vi "Generate Subpanel to Main Event.vi"(8 "error in (no error)":errorcluster, 9 "data":variant, 10 "command":string, 11 "subpanel to main command event":T1) -> (0 "error out":errorcluster)   [LabVIEW 2017, in "NI_Robotics_Configure Steering Frame.lvlib"]
uses:
  <vilib>/robotics/Dialog/Configure Steering Frame/NI_Robotics_Configure Steering Frame.lvlib
  <vilib>/robotics/Dialog/Configure Steering Frame/Subpanel to Main Command Event.ctl
  <vilib>/robotics/Dialog/Configure Steering Frame/Subpanel to Main Command.ctl
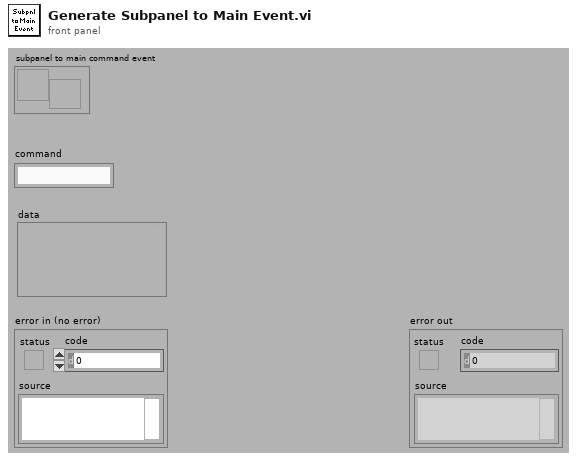
[diagram p1: front panel]
types:
  T1 = typedef "NI_Robotics_Configure Steering Frame.lvlib/Subpanel to Main Command Event.ctl" = refnum<user-event>
  T2 = typedef "NI_Robotics_Configure Steering Frame.lvlib/Subpanel to Main Command.ctl" = cluster{"command":string, "data":variant}
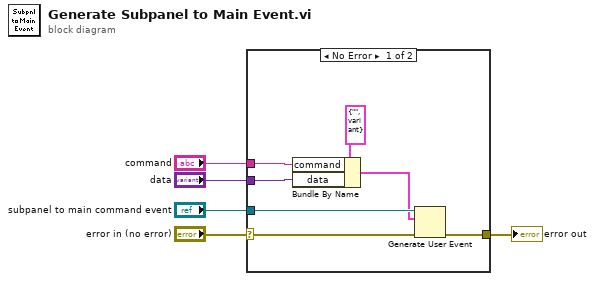
[diagram p0: block diagram]
diagram:
  n1 = case shown="No Error" "error in (no error)" {
    selector: "error in (no error)" -> [w11 w13]
    tunnel: "data" -> [w8 _]
    tunnel: "command" -> [w7 _]
    tunnel: "subpanel to main command event" -> [w12 _]
    tunnel: [w6 w13] -> w1
    frame No Error {
      n2 = Bundle By Name(cluster=T2 {"command"="", "data"=variant} ("subpanel to main command"), "command"=w7, "data"=w8) -> (w9:T2)
      n3 = Generate User Event(user event=w12, event data cluster=w9, error in=w11) -> (error out=w6:errorcluster)  [unwired: 1 in, 1 out]
    }
    frame Error {
    }
  }
  "error out" <- w1
